vi "Scanme.vi"(2 "Index":i32, 4 "Parameters":dbl[](array[numeric]) format="%.3e", 5 "Instrument Address":refnum<visa-resource-name>) -> (0 "Stop":bool, 1 "Array":dbl[](array[numeric]) format="%.2f")   [LabVIEW 2020]
panel:
  in  "max# of channels?":u8=4
  in  "Channel":u8[](array[numeric])=[20, 22, 23, 24, 21, 22, 23, 24]
  out "Command to scanner":string
  # "You are limited to 16 single or 8 double channels"
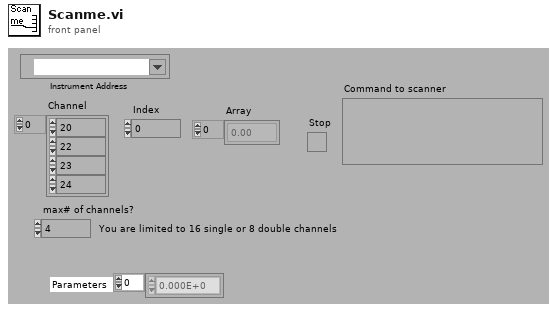
[diagram p1: front panel]
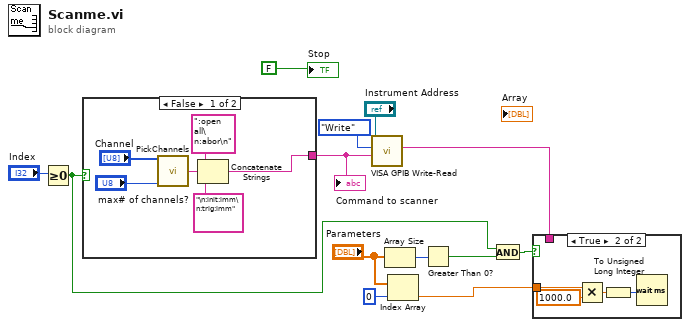
[diagram p0: block diagram]
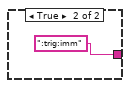
[diagram p3: hidden frame]
diagram:
  n1 = Greater Or Equal To 0?(x="Index") -> (x >= 0?=w5:bool)
  n2 = case shown="False" w5 {
    tunnel: [w19 ":trig:imm"] -> w3
    frame False {
      n3 = call "PickChannels.vi"("# of channels?"="max# of channels?", "Channel"="Channel") -> ("Command"=w16:string)
      n4 = Concatenate Strings(":open all\n:abor\n", w16, "\n:init:imm\n:trig:imm") -> (w19:string)
    }
    frame True {
    }
  }
  "Command to scanner" <- w3
  n5 = call "VISA GPIB Write-Read.vi"("Command"=w3, "Action"=enum16{"Write", "Read", "Write & Read"}."Write", "VISA resource name"="Instrument Address") -> ("String Returned"=w7:string)  [unwired: 5 in, 3 out]
  n6 = Array Size(array="Parameters") -> (size(s)=w9:i32)
  n7 = Index Array(array="Parameters", index=0) -> (element=w11:dbl)
  n8 = Greater Than 0?(x=w9) -> (x > 0?=w6:bool)
  n9 = And(x=w5, y=w6) -> (x .and. y?=w4:bool)
  n10 = case shown="True" w4 {
    tunnel: w7 -> [_ _]
    tunnel: w11 -> [_ w23]
    frame False {
    }
    frame True {
      n11 = Multiply(x=w23, y=1000.0) -> (x*y=w22:dbl)
      n12 = To Unsigned Long Integer(number=w22) -> (unsigned 32bit integer=w21:u32)
      n13 = Wait (ms)(milliseconds to wait=w21) -> ()  [unwired: 1 out]
    }
  }
  "Stop" <- FALSE
